vi "Pre-Process.vi"(11 "Zap Sat in":refnum<class "Zap Sat.lvclass">) -> (3 "Zap Sat out":refnum<class "Zap Sat.lvclass">)   [LabVIEW 2021, in "Zap Sat.lvclass"]
uses:
  Zap Sat.lvclass
  C:/dev/LabVIEW/LabMelee/Source/Application Specific/Element/Element.lvclass
  Element/Element.lvclass/Element.ctl
  Motion/Motion.lvclass/Motion.ctl
  Zap Sat.lvclass/Zap Sat.ctl
  C:/dev/LabVIEW/LabMelee/Source/Application Specific/Deployable/Deployable.lvclass
  C:/dev/LabVIEW/LabMelee/Source/Application Specific/Deployables/Zap Sat/Zap Sat.lvclass
  Element/Element.lvclass
  Motion/Motion.lvclass
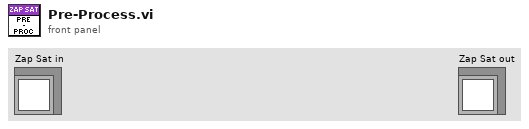
[diagram p1: front panel]
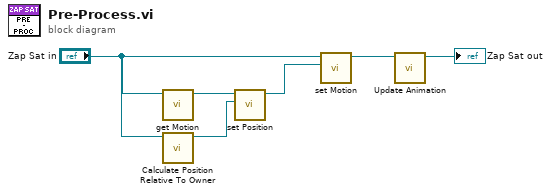
[diagram p0: block diagram]
diagram:
  n1 = call "get Motion.vi"("Element in"="Zap Sat in") -> ("Motion"=w6:refnum<class "Motion.lvclass">)  [unwired: 10 in]
  n2 = call "Calculate Position Relative To Owner.vi"("Zap Sat in"="Zap Sat in") -> ("Position"=w2:refnum<class "Vector 2D.lvclass">)  [unwired: 10 in]
  n3 = call "set Position.vi"("Position"=w2, "Motion in"=w6) -> ("Motion out"=w5:refnum<class "Motion.lvclass">)  [unwired: 9 in]
  n4 = call "set Motion.vi"("Motion"=w5, "Element in"="Zap Sat in") -> ("Element out"=w4:refnum<class "Zap Sat.lvclass">)  [unwired: 9 in]
  n5 = call "Update Animation.vi"("Deployable in"=w4) -> ("Deployable out"=→"Zap Sat out":refnum<class "Zap Sat.lvclass">)  [unwired: 10 in]
